vi "Shutter.vi"() -> ()   [LabVIEW 2018]
uses:
  <vilib>/DAQmx/write.llb/DAQmx Write (Digital Bool 1Line 1Point).vi
  <vilib>/DAQmx/create/channels.llb/DAQmx Create Channel (DO-Digital Output).vi
  <vilib>/DAQmx/miscellaneous.llb/DAQmx Fill In Error Info.vi
  <resource>/objmgr/daqmx.rc
panel:
  in  "Mode":enum16{"Manual", "Auto"}(ring)
  in  "Shutter open":bool
  in  "DAQmx Device Name":tag="Voltage_PXIe"
  in  "milliseconds to wait":u32=1000
  in  "Line Number":i32=8
  in  "stop":bool
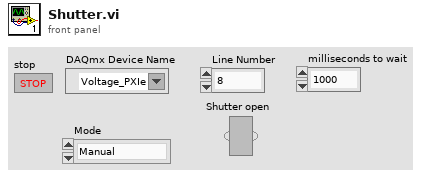
[diagram p1: front panel]
types:
  T1 = enum16{"open", "open or create", "create or replace", "create", "open (read-only)"}
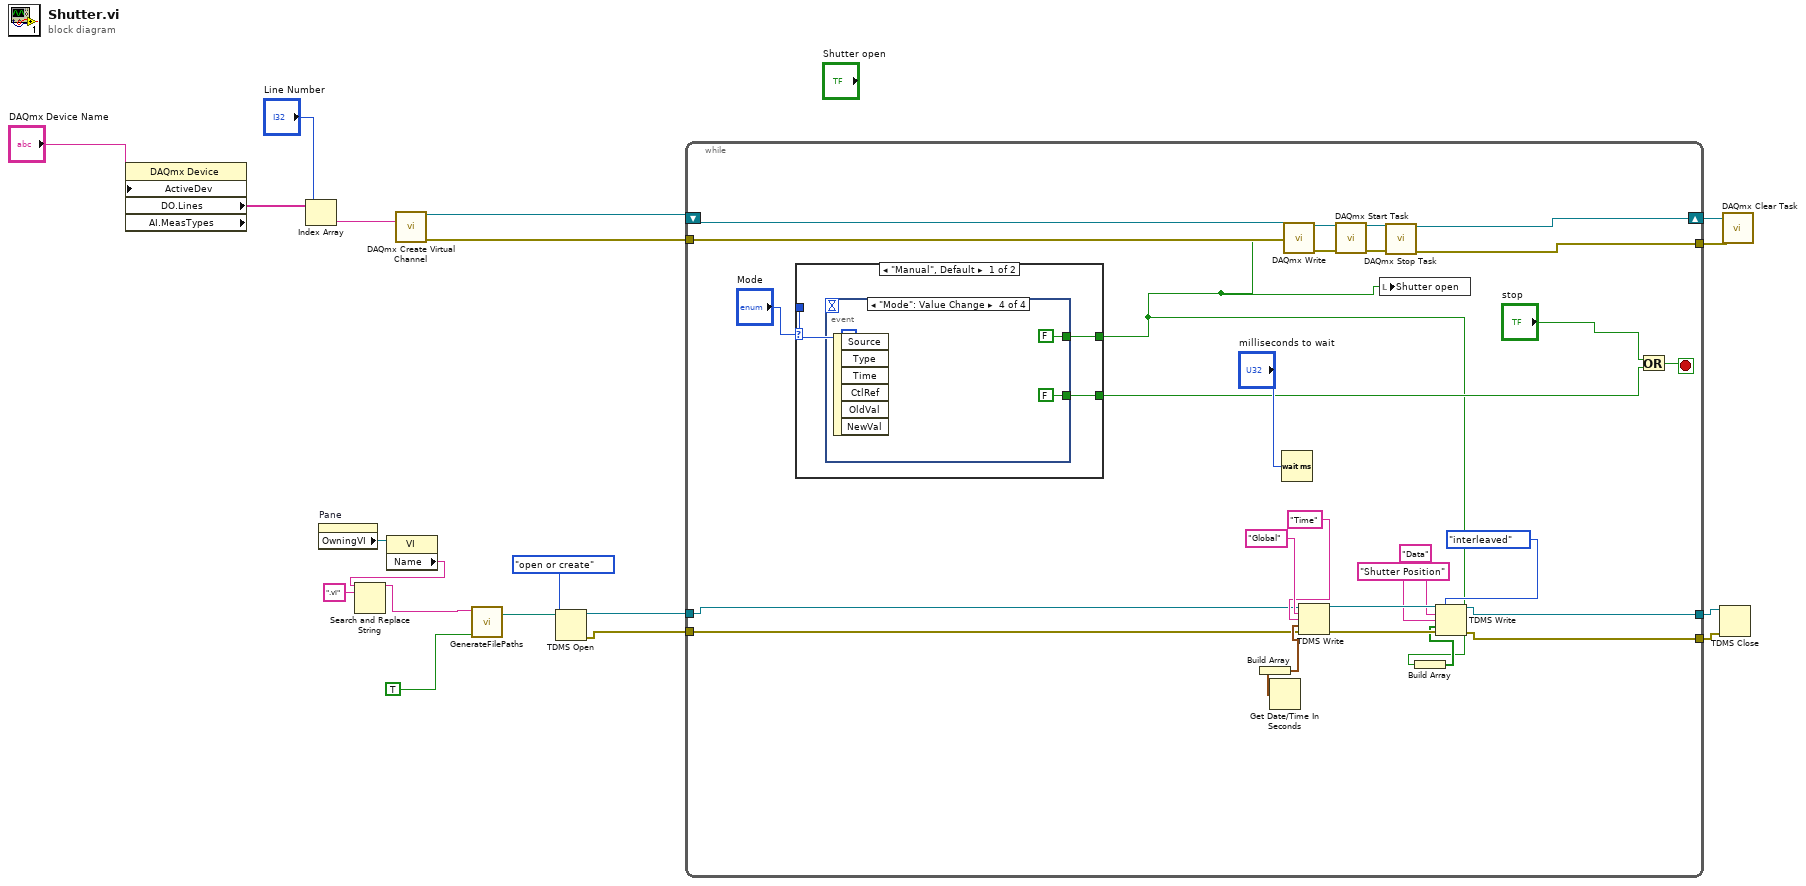
[diagram p0: block diagram]
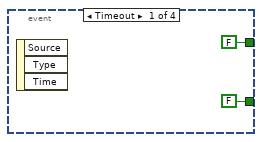
[diagram p2: hidden frame]
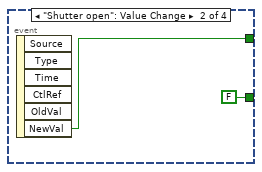
[diagram p3: hidden frame]
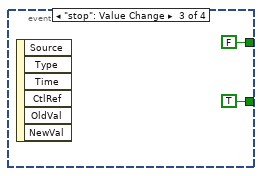
[diagram p4: hidden frame]
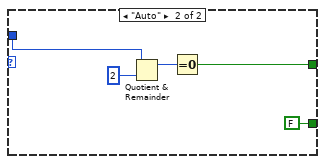
[diagram p5: hidden frame]
diagram:
  n1 = property class="DAQmx Device" props=["ActiveDev", "DO.Lines", "AI.MeasTypes"]("ActiveDev"="DAQmx Device Name") -> ("DO.Lines"=w18:tag[])  [unwired: 2 in, 3 out]
  n2 = Index Array(array=w18, index="Line Number") -> (element=w17:tag)
  n3 = property on="Pane" class="Pane"() -> ("OwningVI"=w11:refnum<vi>)  [unwired: 2 in, 2 out]
  n4 = property class="VI"(reference=w11) -> ("Name"=w5:string)  [unwired: 1 in, 2 out]
  n5 = Search and Replace String(input string=w5, search string=".vi") -> (result string=w9:string)  [unwired: 6 in, 3 out]
  n6 = call-poly <vilib>:"DAQmx Create Virtual Channel.vi"("lines"=w17) -> ("task out"=w16:refnum<k21>, "error out"=w13:errorcluster)  [unwired: 13 in]
  n7 = call "GenerateFilePaths.vi"("Logfile? (F)"=TRUE ("Logfile?"), "Device Name"=w9) -> ("Path"=w7:path)  [unwired: 3 in]
  n8 = TDMS Open(10:T1."open or create" ("operation (0:open)"), 11:w7) -> (0:w3:errorcluster, 3:w4:refnum<k34>)  [unwired: 5 in]
  n9 = while {
    shift-right: [w43] -> w15
    shift-left: w16 -> [w48]
    tunnel: [w42] -> w14
    tunnel: w13 -> [w41]
    tunnel: w4 -> [w31]
    tunnel: w3 -> [w30]
    tunnel: [w26] -> w1
    tunnel: [w25] -> w2
    i -> [w40]
    stop <- w23 stop-if-true
    n10 = case shown="\"Manual\", Default" "Mode" {
      tunnel: w40 -> [_ w63]
      tunnel: [w50 w60] -> w20
      tunnel: [w49 FALSE ("NewVal")] -> w21
      frame "Manual", Default {
        n11 = event shown="[3] \"Mode\": Value Change" {
          selector: _ -> [_ _ _ _]
          dyn-events: _ -> [_ _ _ _]
          timeout: _ -> [_ _ _ _]
          tunnel: [FALSE ("NewVal") w54 FALSE ("NewVal") FALSE ("NewVal")] -> w50
          tunnel: [FALSE ("NewVal") FALSE ("NewVal") TRUE ("NewVal") FALSE ("NewVal")] -> w49
          event Timeout {
            n12 = event-data() -> ()  [unwired: 1 in, 3 out]
          }
          event "Shutter open": Value Change {
            n13 = event-data() -> ("NewVal"=w54:bool)  [unwired: 1 in, 5 out]
          }
          event "stop": Value Change {
            n14 = event-data() -> ()  [unwired: 1 in, 6 out]
          }
          event "Mode": Value Change {
            n15 = event-data() -> ()  [unwired: 1 in, 6 out]
          }
        }
      }
      frame "Auto" {
        n16 = Quotient & Remainder(x=w63, y=2) -> (x-y*floor(x/y)=w61:i32)  [unwired: 1 out]
        n17 = Equal To 0?(x=w61) -> (x = 0?=w60:bool)
      }
    }
    n18 = Get Date/Time In Seconds() -> (seconds since 1Jan1904=w35:timestamp)
    n19 = Build Array(w35) -> (w36:timestamp[])
    n20 = Wait (ms)(milliseconds to wait="milliseconds to wait") -> ()  [unwired: 1 out]
    n21 = call-poly <vilib>:"DAQmx Write.vi"("task/channels in"=w48, "data"=w20, "error in"=w41) -> ("task out"=w47:refnum<k21>, "error out"=w46:errorcluster)  [unwired: 10 in, 1 out]
    n22 = TDMS Write(0:w31, 5:"Global" ("group name in (Untitled)"), 7:"Time" ("group name in (Untitled)"), 9:w36, 11:w30) -> (4:w37:refnum<k34>, 15:w38:errorcluster)  [unwired: 1 in, 2 out]
    n23 = call <vilib>:"DAQmx Start Task.vi"("task/channels in"=w47, "error in"=w46) -> ("task out"=w45:refnum<k21>, "error out"=w44:errorcluster)  [unwired: 12 in]
    n24 = local write "Shutter open"(w20) -> ()
    n25 = call <vilib>:"DAQmx Stop Task.vi"("task/channels in"=w45, "error in"=w44) -> ("task out"=w43:refnum<k21>, "error out"=w42:errorcluster)  [unwired: 12 in]
    n26 = Build Array(w20) -> (w29:bool[])
    n27 = TDMS Write(0:w37, 1:enum16{"decimated", "interleaved"}."interleaved" ("data layout (0:decimated)"), 5:"Data" ("group name in (Untitled)"), 7:"Shutter Position" ("group name in (Untitled)"), 9:w29, 11:w38) -> (4:w26:refnum<k34>, 15:w25:errorcluster)  [unwired: 2 out]
    n28 = Or(x="stop", y=w21) -> (x .or. y?=w23:bool)
  }
  n29 = TDMS Close(8:w2, 11:w1) -> ()  [unwired: 2 out]
  n30 = call <vilib>:"DAQmx Clear Task.vi"("task in"=w15, "error in"=w14) -> ()  [unwired: 13 in, 1 out]
